vi "Load and Open All Items.vi"(8 "error in (no error)":errorcluster, 11 "Application Data in":T1) -> (0 "error out":errorcluster, 3 "Application Data out":T1)   [LabVIEW 2017, in "DSF Data Viewer.lvlib"]
uses:
  DSF Data Viewer.lvlib
  Application Data.ctl
  Builds/Data Sharing Framework/Current/Core/DSF Core.lvlibp/Engine/Classes/Framework/Framework.lvclass
  <vilib>/NI/Memory Manager/Classes/Pointer/Pointer.lvclass
  Buffer Reader/Buffer Data.ctl
  Builds/Data Sharing Framework/Current/Core/DSF Core.lvlibp/Engine/Classes/Buffer/Buffer.lvclass
  Item Tree/Create Plugins.vi
  Item Tree/Add Plugin with Children.vi
  Item Tree/Create New Tree Item.vi
  Item Tree/Add Transfer Group with Children.vi
  Item Tree/Add Buffer Data to Variant.vi
  Item Tree/Add Transfer.vi
  Item Tree/Add Buffers.vi
  Set UI Busy State.vi
  Item Tree/Add Item to Tree.vi
  Builds/Data Sharing Framework/Current/Core/DSF Core.lvlibp/Engine/Classes/Buffer/Get String Buffer.vi
  Builds/Data Sharing Framework/Current/Core/DSF Core.lvlibp/Engine/Classes/Buffer/Get Async Buffer.vi
  Builds/Data Sharing Framework/Current/Core/DSF Core.lvlibp/Engine/Classes/Buffer/Get Inline Buffer.vi
  Builds/Data Sharing Framework/Current/Core/DSF Core.lvlibp/Engine/Classes/Transfer/Get Buffers.vi
  Builds/Data Sharing Framework/Current/Core/DSF Core.lvlibp/Engine/Classes/Transfer/Get Name.vi
  Builds/Data Sharing Framework/Current/Core/DSF Core.lvlibp/Engine/Classes/Timing/Get Decimation.vi
  Builds/Data Sharing Framework/Current/Core/DSF Core.lvlibp/Engine/Classes/Transfer Group/Get Inline.vi
  Builds/Data Sharing Framework/Current/Core/DSF Core.lvlibp/Engine/Classes/Transfer Group/Get Transfers.vi
  Builds/Data Sharing Framework/Current/Core/DSF Core.lvlibp/Engine/Classes/Transfer Group/Get Timing.vi
  Builds/Data Sharing Framework/Current/Core/DSF Core.lvlibp/Engine/Classes/Transfer Group/Get Name.vi
  Builds/Data Sharing Framework/Current/Core/DSF Core.lvlibp/Engine/Classes/Plugin/Get Name.vi
  Builds/Data Sharing Framework/Current/Core/DSF Core.lvlibp/Engine/Classes/Plugin/Get Async Rx Transfer Groups.vi
  Builds/Data Sharing Framework/Current/Core/DSF Core.lvlibp/Engine/Classes/Plugin/Get Async Tx Transfer Groups.vi
  Builds/Data Sharing Framework/Current/Core/DSF Core.lvlibp/Engine/Classes/Plugin/Get Inline Rx Transfer Groups.vi
  Builds/Data Sharing Framework/Current/Core/DSF Core.lvlibp/Engine/Classes/Plugin/Get Inline Tx Transfer Groups.vi
  Builds/Data Sharing Framework/Current/Core/DSF Core.lvlibp/Engine/Classes/Plugin/Get Buffers.vi
  Builds/Data Sharing Framework/Current/Core/DSF Core.lvlibp/Engine/Classes/Plugin/Get Timing.vi
  Builds/Data Sharing Framework/Current/Core/DSF Core.lvlibp/Engine/Classes/Framework/Get Async Plugins.vi
  Builds/Data Sharing Framework/Current/Core/DSF Core.lvlibp/Engine/Classes/Framework/Get Inline Plugins.vi
  Initialize Tree.vi
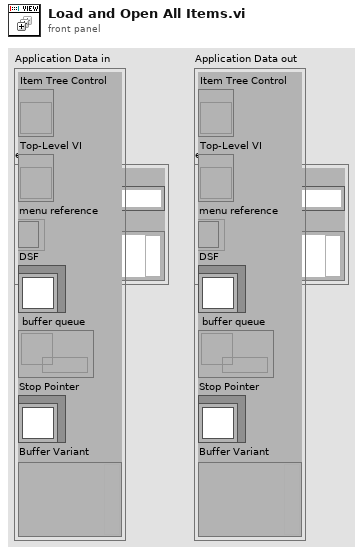
[diagram p1: front panel]
types:
  T1 = typedef "DSF Data Viewer.lvlib/Application Data.ctl" = cluster{"Item Tree Control":refnum<vi>, "Top-Level VI":refnum<vi>, "menu reference":refnum<k9>, "DSF":refnum<class "Framework.lvclass">, "buffer queue":refnum<queue>, "Stop Pointer":refnum<class "Pointer.lvclass">, "Buffer Variant":variant}
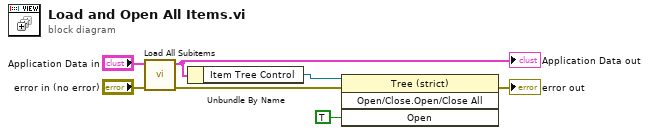
[diagram p0: block diagram]
diagram:
  n1 = call "Load All Subitems.vi"("error in (no error)"="error in (no error)", "Application Data in"="Application Data in") -> ("error out"=w1:errorcluster, "Application Data out"=w4:T1)  [unwired: 8 in]
  "Application Data out" <- w4
  n2 = Unbundle By Name(w4) -> ("Item Tree Control"=w6:refnum<vi>)
  n3 = invoke class="Tree (strict)" method="Open/Close.Open/Close All"(reference=w6, error in=w1, "Open"=TRUE ("Open?")) -> (error out=→"error out":errorcluster)  [unwired: 1 in, 3 out]
